vi "Rotate Around a Point.vi"(5 "Y Center Pixel":i32=21, 6 "Angle (degrees)":sgl format="%.2f", 7 "X Center Pixel":i32=21, 8 "Y Pixel":i32=34, 9 "X Pixel":i32=21, 10 "Image Dst":T1, 11 "Image Src":T1) -> (3 "Image Dst Out":T1)   [LabVIEW 2013]
doc: "This VI should take an image, an angle, and a point to rotate the image around, then it should rotate the image around that point. This VI rotates around a point by putting the point at the center, rotating the image, and shifting the point back. Filler color is black\n\nEric Schneider, June 2014"
uses:
  <vilib>/vision/Image Controls.llb/IMAQ Image.ctl
  <vilib>/vision/NI_Vision_Development_Module.lvlib
panel:
  out "Image out display":T1(plugin-control)
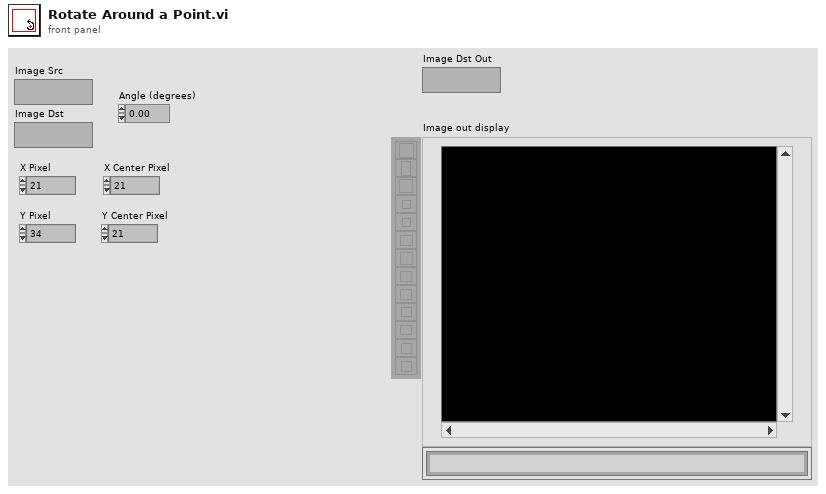
[diagram p1: front panel]
types:
  T1 = typedef "IMAQ Image.ctl" = refnum<image>
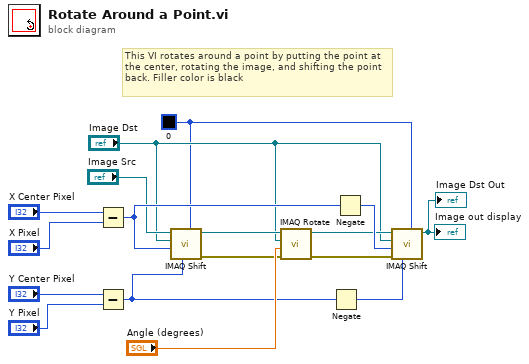
[diagram p0: block diagram]
diagram:
  w1 = u32 0 ("Color Replace Value")
  # "This VI rotates around a point by putting the point at the center, rotating the image, and shifting the point back. Filler color is black"
  n1 = Subtract(x="X Center Pixel", y="X Pixel") -> (x-y=w10:i32)
  n2 = Subtract(x="Y Center Pixel", y="Y Pixel") -> (x-y=w8:i32)
  n3 = call "IMAQ Shift"("Color Replace Value"=w1, "YOffset"=w8, "XOffset"=w10, "Image Dst"="Image Dst", "Image Src"="Image Src") -> ("error out"=w6:errorcluster, "Image Dst Out"=w4:T1)  [unwired: 5 in]
  n4 = call "IMAQ Rotate"("error in (no error)"=w6, "Angle (degrees)"="Angle (degrees)", "Image Dst"="Image Dst", "Image Src"=w4) -> ("error out"=w17:errorcluster, "Image Dst Out"=w5:T1)  [unwired: 6 in]
  n5 = Negate(x=w8) -> (-x=w7:i32)
  n6 = Negate(x=w10) -> (-x=w9:i32)
  n7 = call "IMAQ Shift"("Color Replace Value"=w1, "YOffset"=w7, "error in (no error)"=w17, "XOffset"=w9, "Image Dst"="Image Dst", "Image Src"=w5) -> ("Image Dst Out"=→"Image Dst Out" →"Image out display":T1)  [unwired: 4 in, 1 out]
